vi "Read receivedTimeStamp.vi"(8 "error in (no error)":errorcluster, 11 "RobotFeedback in":refnum<class "RobotFeedback.lvclass">) -> (0 "error out":errorcluster, 2 "receivedTimeStamp":timestamp, 3 "RobotFeedback out":refnum<class "RobotFeedback.lvclass">)   [LabVIEW 2021, in "RobotFeedback.lvclass"]
uses:
  RobotFeedback.lvclass
  RobotFeedback.lvclass/RobotFeedback.ctl
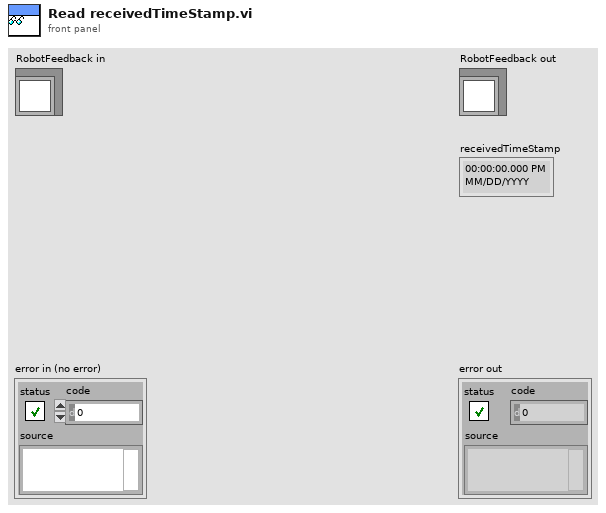
[diagram p1: front panel]
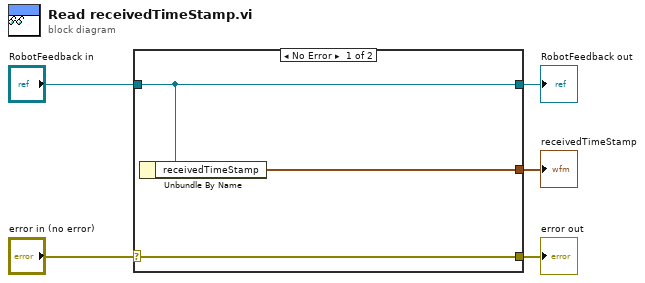
[diagram p0: block diagram]
diagram:
  n1 = case shown="No Error" "error in (no error)" {
    selector: "error in (no error)" -> [w8 w9]
    tunnel: [w8 w9] -> w4
    tunnel: [w7 w10] -> w2
    tunnel: "RobotFeedback in" -> [w7 w10]
    tunnel: [w6 _] -> w1
    frame No Error {
      n2 = Unbundle By Name(w7) -> ("receivedTimeStamp"=w6:timestamp)
    }
    frame Error {
    }
  }
  "error out" <- w4
  "RobotFeedback out" <- w2
  "receivedTimeStamp" <- w1
